vi "ATE_Test_Pulse_2.vi"() -> ()   [LabVIEW 2009]
doc: "Use this template to build a producer/consumer design pattern with events to produce queue items. Use this design pattern instead of the User Interface Event Handler pattern for user interfaces when you want to execute code asynchronously in response to an event without slowing the user interface responsiveness."
panel:
  in  "exit":bool
  in  "ATE TP TABS":T1(tab)
  in  "Signal Generator Control":T2={"Frequency (GHz)"=2.809, "RF Power (dBm)"=-120.0, "RF ON/OFF"=FALSE} {"RF Power (dBm)" min=-120.0 max=20.0 step=5.0 format="%.2g"; "Frequency (GHz)" min=0.6 max=3.0 step=0.001 format="%#_9g"}
  out "Signal Generator Status":T3={"Frequency (GHz)"=2.809, "RF Power (dBm)"=-120.0, "RF Power"=FALSE} {"RF Power (dBm)" format="%.2g"}
  out "Switch Position\nVerfied":bool
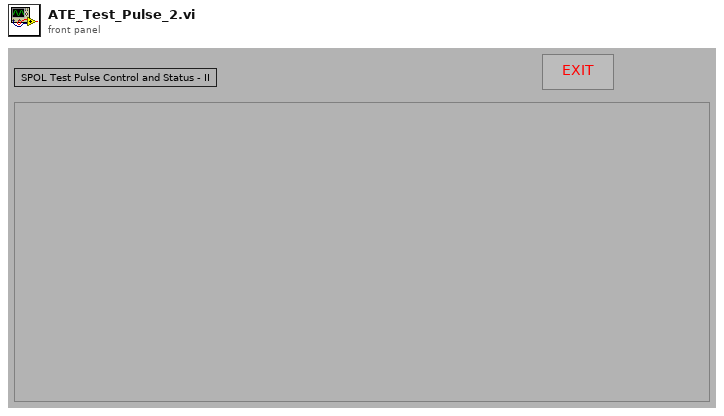
[diagram p1: front panel]
types:
  T1 = enum32{"SPOL Test Pulse Control and Status - II"}
  T2 = cluster{"Frequency (GHz)":dbl, "RF Power (dBm)":dbl, "RF ON/OFF":bool}
  T3 = cluster{"Frequency (GHz)":dbl, "RF Power (dBm)":dbl, "RF Power":bool}
  T4 = enum16{"NONE", "Amp Bypass Switch", "Test Pulse Generator", "Power Meter Switch (S5)"}
  T5 = enum16{"NONE", "Delay Device", "Signal Generator (J7)", "Inside Noise Box NF (J5)", "2W Term (TM3)"}
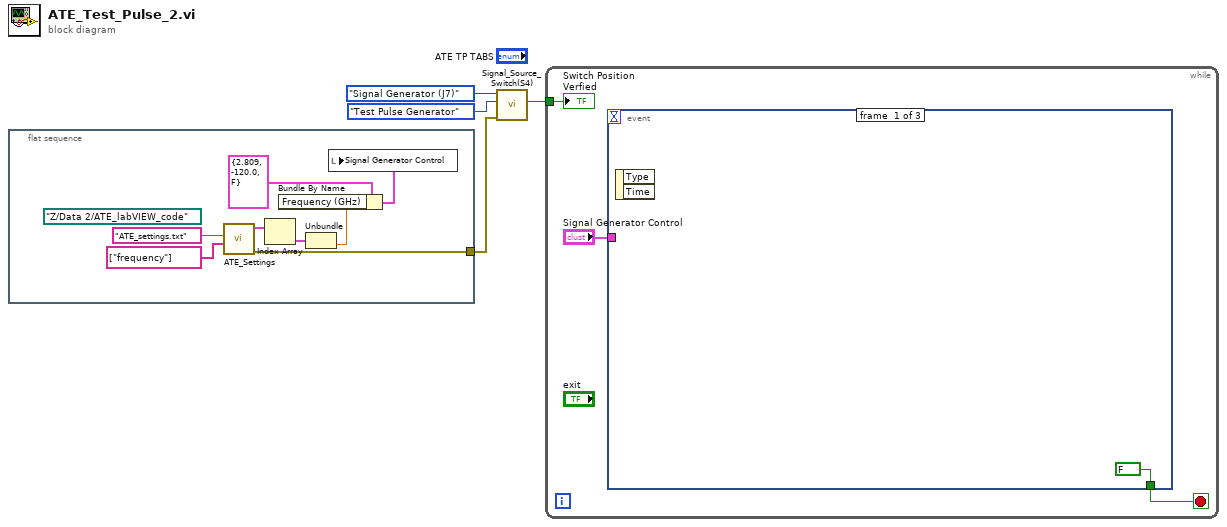
[diagram p0: block diagram]
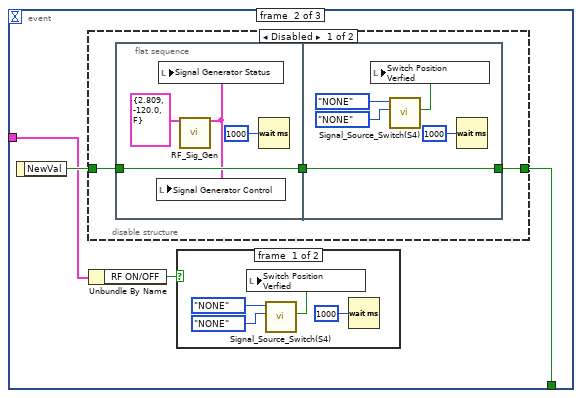
[diagram p2: hidden frame]
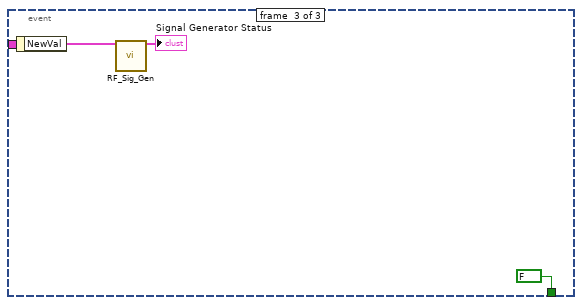
[diagram p5: hidden frame]
diagram:
  n1 = flat-sequence {
    tunnel: [w5] -> w1
    frame #0 {
      (unwired) path "Z:/Data 2/ATE_labVIEW_code" ("start path")
      n2 = call "ATE_Settings.vi"("Variable to Read"=string[] ["frequency"], "file name"="ATE_settings.txt") -> ("error out"=w5:errorcluster, "NewVariables"=w10:cluster{"Name":string, "Value":dbl}[])  [unwired: 8 in]
      n3 = Index Array(array=w10) -> (element=w9:cluster{"Name":string, "Value":dbl})  [unwired: 1 in]
      n4 = Unbundle(w9) -> ("Value"=w7:dbl)  [unwired: 1 out]
      n5 = Bundle By Name(cluster=T2 {"Frequency (GHz)"=2.809, "RF Power (dBm)"=-120.0, "RF ON/OFF"=FALSE} ("Signal Generator Control"), "Frequency (GHz)"=w7) -> (w6:T2)
      n6 = local write "Signal Generator Control"(w6) -> ()
    }
  }
  n7 = call "Signal_Source_Switch(S4).vi"("error in"=w1, "Output"=T4."Test Pulse Generator" ("ATE Switch (S4) Output"), "Input"=T5."Signal Generator (J7)" ("ATE Switch (S4) Input")) -> ("Verfied"=w2:bool)  [unwired: 6 in, 2 out]
  n8 = while {
    tunnel: w2 -> [w14]
    stop <- w15 stop-if-true
    n9 = event shown="[1] \"exit\": Value Change" {
      selector: _ -> [_ _ _]
      dyn-events: _ -> [_ _ _]
      timeout: _ -> [_ _ _]
      tunnel: [FALSE w20 FALSE] -> w15
      tunnel: "Signal Generator Control" -> [_ w18 _]
      event #0 {
        n10 = event-data() -> ()  [unwired: 1 in, 2 out]
      }
      event #1 {
        n11 = event-data() -> ("NewVal"=w19:bool)  [unwired: 1 in]
        n12 = disable-structure shown="Disabled" {
          disable-tunnel: [w26 w37] -> w20
          disable-tunnel: w19 -> [w25 w37]
          frame #0 {
            n13 = flat-sequence {
              tunnel: w25 -> [w29]
              tunnel: [w29] -> w27
              tunnel: [w32] -> w26
              tunnel: w27 -> [w32]
              frame #0 {
                n14 = call "RF_Sig_Gen.vi"("Signal Generator Control"=T2 {"Frequency (GHz)"=2.809, "RF Power (dBm)"=-120.0, "RF ON/OFF"=FALSE}) -> ("Signal Generator Status"=w28:T3)  [unwired: 13 in, 1 out]
                n15 = local write "Signal Generator Control"(w28) -> ()
                n16 = local write "Signal Generator Status"(w28) -> ()
                n17 = Wait (ms)(milliseconds to wait=u32 1000) -> ()  [unwired: 1 out]
              }
              frame #1 {
                n18 = call "Signal_Source_Switch(S4).vi"("Output"=T4."NONE" ("ATE Switch (S4) Output"), "Input"=T5."NONE" ("ATE Switch (S4) Input")) -> ("Verfied"=w36:bool)  [unwired: 7 in, 2 out]
                n19 = local write "Switch Position\nVerfied"(w36) -> ()
                n20 = Wait (ms)(milliseconds to wait=u32 1000) -> ()  [unwired: 1 out]
              }
            }
          }
          frame #1 {
          }
        }
        n21 = Unbundle By Name(w18) -> ("RF ON/OFF"=w17:bool)
        n22 = case shown="False" w17 {
          frame #0 {
            n23 = call "Signal_Source_Switch(S4).vi"("Output"=T4."NONE" ("ATE Switch (S4) Output"), "Input"=T5."NONE" ("ATE Switch (S4) Input")) -> ("Verfied"=w21:bool)  [unwired: 7 in, 2 out]
            n24 = local write "Switch Position\nVerfied"(w21) -> ()
            n25 = Wait (ms)(milliseconds to wait=u32 1000) -> ()  [unwired: 1 out]
          }
          frame #1 {
          }
        }
      }
      event #2 {
        n26 = event-data() -> ("NewVal"=w39:T2)  [unwired: 1 in]
        n27 = call "RF_Sig_Gen.vi"("Signal Generator Control"=w39) -> ("Signal Generator Status"=→"Signal Generator Status":T3)  [unwired: 13 in, 1 out]
      }
    }
    "Switch Position\nVerfied" <- w14
  }
